vi "I64 to I32.vi"(2 "error in (no error)":errorcluster, 3 "I64":dbl) -> (0 "error out":errorcluster, 1 "I32":i32)   [LabVIEW 2017]
panel:
  # "LVHDF5 Toolkit\nCopyright (c) 2005-2013 by Jason D. Sommerville\nCopyright (c) 2014 by UPVI, LLC.\n\nThis use and distribution of this file is governed by the terms found in \nLICENSE.txt distributed with this toolkit and installed at\n <user.lib>\\_lvhdf5\\LICENSE.txt"
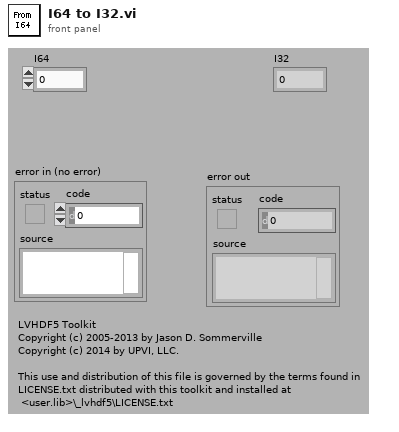
[diagram p1: front panel]
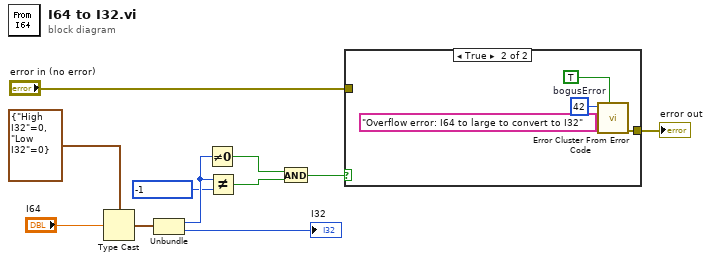
[diagram p0: block diagram]
diagram:
  n1 = Type Cast(type=cluster{"High I32":i32, "Low I32":i32} {"High I32"=0, "Low I32"=0}, x="I64") -> (*(type *) &x=w9:cluster{"High I32":i32, "Low I32":i32})
  n2 = Unbundle(w9) -> ("High I32"=w3:i32, "Low I32"=→"I32":i32)
  n3 = Not Equal To 0?(x=w3) -> (x != 0?=w4:bool)
  n4 = Not Equal?(x=w3, y=-1) -> (x != y?=w1:bool)
  n5 = And(x=w4, y=w1) -> (x .and. y?=w5:bool)
  n6 = case shown="True" w5 {
    tunnel: [w12 w13] -> w8
    tunnel: "error in (no error)" -> [w12 _]
    frame False {
    }
    frame True {
      w16 = 42  # bogusError
      n7 = call <vilib>:"Error Cluster From Error Code.vi"("show call chain? (False)"=TRUE, "error message (\"\")"="Overflow error: I64 to large to convert to I32" ("error message (\"\")"), "error code (0)"=w16) -> ("error out"=w13:errorcluster)  [unwired: 6 in]
    }
  }
  "error out" <- w8
